vi "Add Styles.vi"(8 "error in (no error)":errorcluster, 10 "Styles":T1[](array[typedef]), 11 "Nav Route in":refnum<class "Nav Route.lvclass">) -> (0 "error out":errorcluster, 3 "Nav Route out":refnum<class "Nav Route.lvclass">)   [LabVIEW 2020, in "Volatus.lvlib" / "Nav Route.lvclass"]
uses:
  Nav Route.lvclass
  Nav Route.lvclass/Nav Route.ctl
  Style.ctl
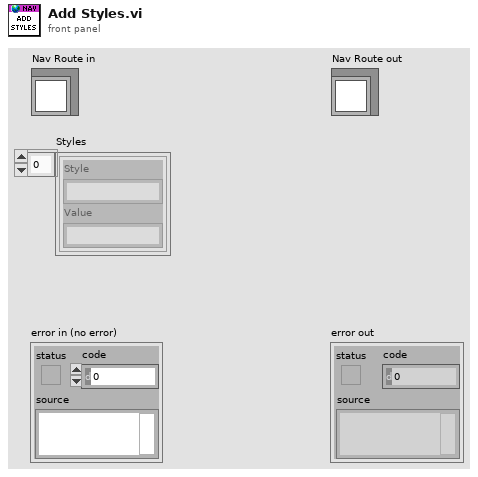
[diagram p1: front panel]
types:
  T1 = typedef "Volatus.lvlib/Nav Route.lvclass/Style.ctl" = cluster{"Style":string, "Value":string}
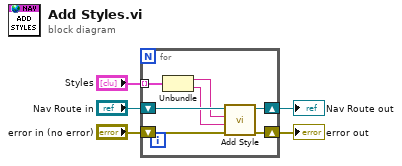
[diagram p0: block diagram]
diagram:
  n1 = for {
    shift-right: [w11] -> w4
    shift-left: "error in (no error)" -> [w12]
    shift-right: [w9] -> w2
    shift-left: "Nav Route in" -> [w10]
    tunnel: "Styles" -> [w8] mode=indexing
    n2 = Unbundle(w8) -> ("Style"=w6:string, "Value"=w7:string)
    n3 = call "Add Style.vi"("error in (no error)"=w12, "Value"=w7, "Style"=w6, "Nav Route in"=w10) -> ("error out"=w11:errorcluster, "Nav Route out"=w9:refnum<class "Nav Route.lvclass">)  [unwired: 6 in]
  }
  "error out" <- w4
  "Nav Route out" <- w2
